vi "NiPxi6733.vi"() -> ()   [LabVIEW 2018, in "Visualization.lvlib" / "VisualizeFGen.lvclass"]
doc: "This VI listens for any measurement data associated with the provided PluginName and displays it to the user for analysis. The display is only suitable for data coming from the RoomAlert Plugin."
uses:
  VisualizeFGen.lvclass
  <vilib>/event_ctls.llb/usereventprio.ctl
  VisualizeBase/VisualizeBase_class/Requests/VisUserEventType.ctl
  <extravilib>/ChannelInstances/Tag-bool/Write With Abort.vi
  <extravilib>/ChannelInstances/Tag-bool/Read With Abort.vi
  <extravilib>/ChannelInstances/Tag-bool/Instantiate.vi
  <extravilib>/ChannelInstances/Tag-bool/EndpointRead.vi
  <vilib>/Utility/error.llb/Error Cluster From Error Code.vi
  <extravilib>/ChannelInstances/Tag-bool/Endpoint.vi
  <vilib>/ErrorRing/Error Ring.xnode
  <userlib>/NIST/NISTErrorLib/NISTErrorLib.lvlib
  <extravilib>/ChannelInstances/Tag-bool.lvlib
  TestClass/Test.lvclass
  VisualizeBase/VisualizeBase_class/VisualizeBase.lvclass
  FGen/FgenShared/FgenShared.lvlib
panel:
  in  "btnPause":bool=TRUE
  in  "ModuleID":i32
  in  "Log Data":bool
  in  "btnStop":bool
  in  "btnReset":bool
  in  "btnClearTest":bool
  out "WfrmGraph":waveform(dbl)[](graph)=[{"t0"=timestamp(3657200531.6397257 s since 1904-01-01), "dt"=1.0, "Y"=[46.19]}, {"t0"=timestamp(3657200531.6397257 s since 1904-01-01), "dt"=1.0, "Y"=[2.0]}, {"t0"=timestamp(3657200531.6397257 s since 1904-01-01), "dt"=1.0, "Y"=[60.0]}]
  out "ErrorArray":errorcluster[](array[cluster])
  in  "PluginName":string="Sensor.RoomAlert1"
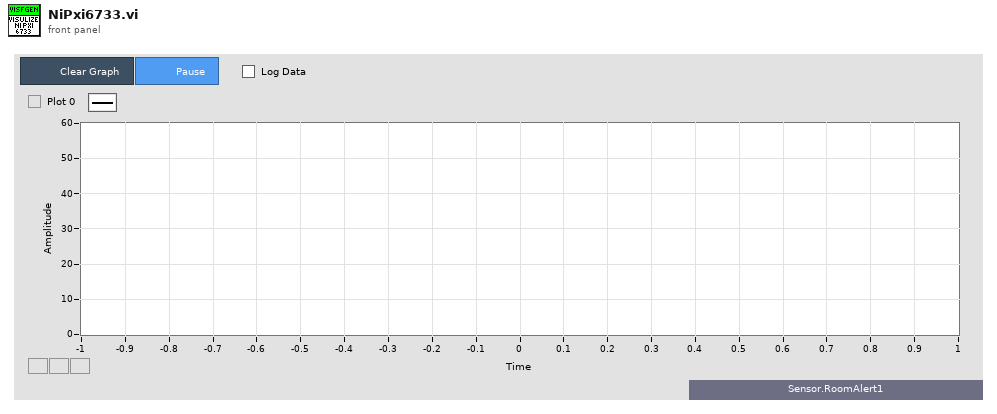
[diagram p1: front panel]
types:
  T1 = enum16{"open", "open or create", "create or replace", "create", "open (read-only)"}
  T2 = typedef "Visualization.lvlib/VisualizeBase.lvclass/VisRequestEvents.ctl" = cluster{"StopRequest":refnum<user-event>, "ResetRequest":refnum<user-event>, "FP Pop In or Out":refnum<user-event>}
  T3 = typedef "FgenShared.lvlib/clBroadcastEvents.ctl" = cluster{"DidInit":refnum<user-event>, "StatusUpdate":refnum<user-event>, "ErrorReport":refnum<user-event>, "DidStop":refnum<user-event>, "PathToINI":refnum<user-event>, "Channels":refnum<user-event>, "Function":refnum<user-event>, "Waveforms":refnum<user-event>, "Triggers":refnum<user-event>, "FunctionParams":refnum<user-event>, "FunctionArbs":refnum<user-event>, "FunctionSampleRate":refnum<user-event>}
  T4 = typedef "Visualization.lvlib/VisualizeBase.lvclass/VisUserEventType.ctl" = cluster{"BusIndex":i8, "Data":variant}
  T5 = typedef "usereventprio.ctl" = enum32{"high priority", "normal priority"}
  T6 = typedef "Tag-bool.lvlib/))Channel.ctl" = refnum<queue>
  T7 = typedef "sizeaction.ctl" = enum32{"Minimized", "Maximized", "Resized"}
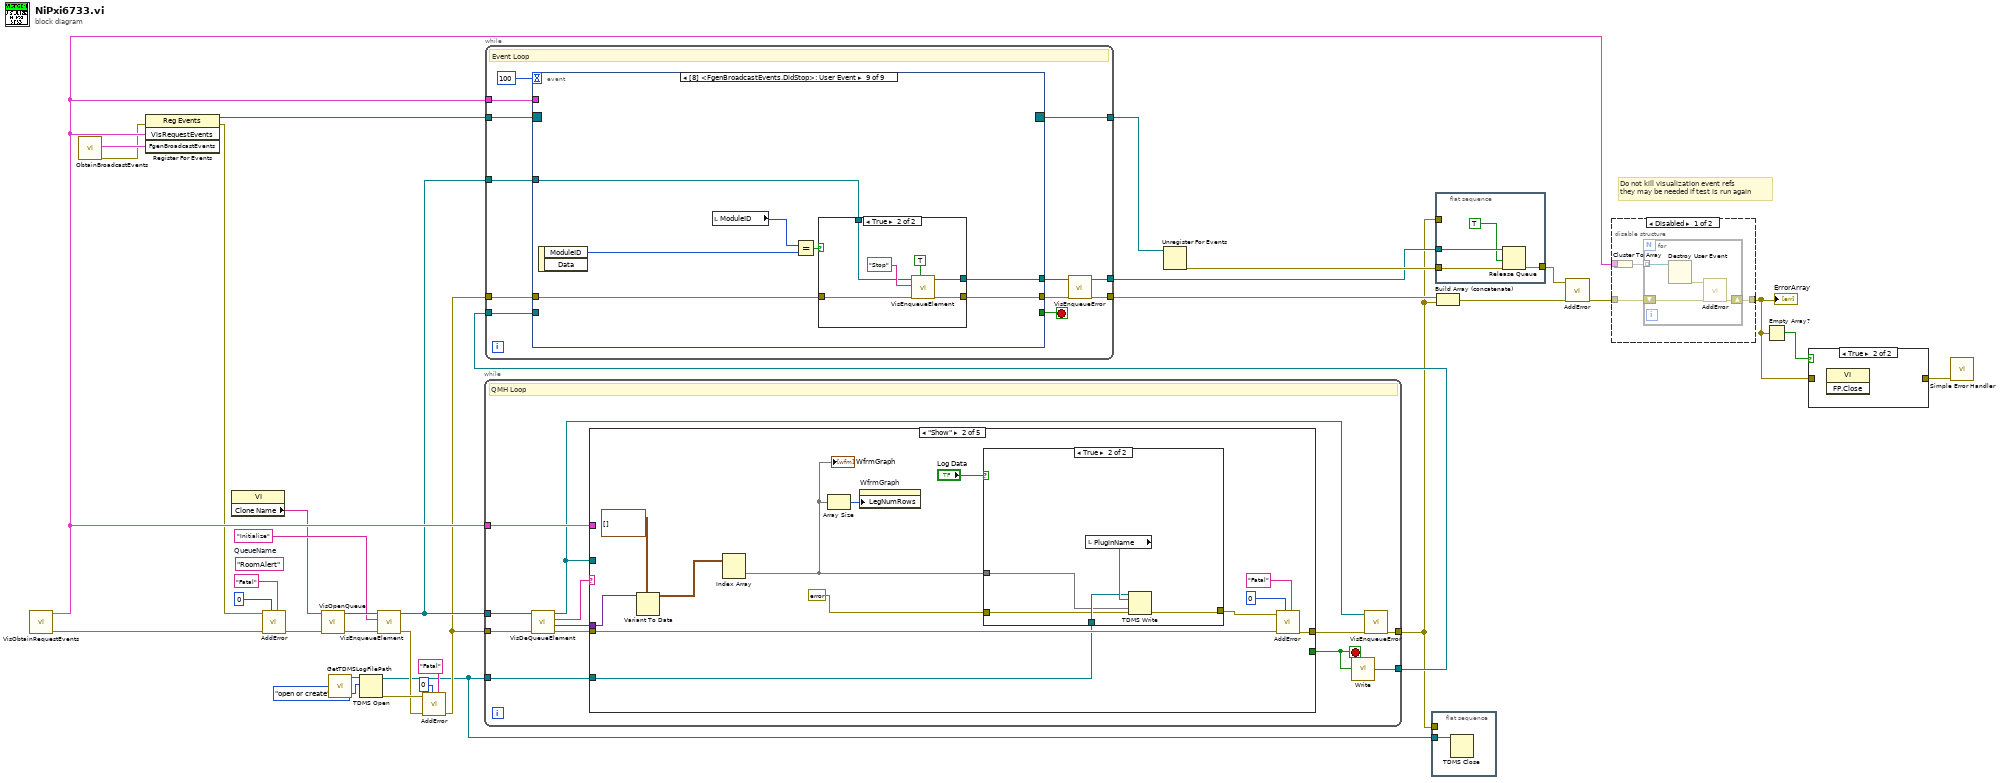
[diagram p0: block diagram]
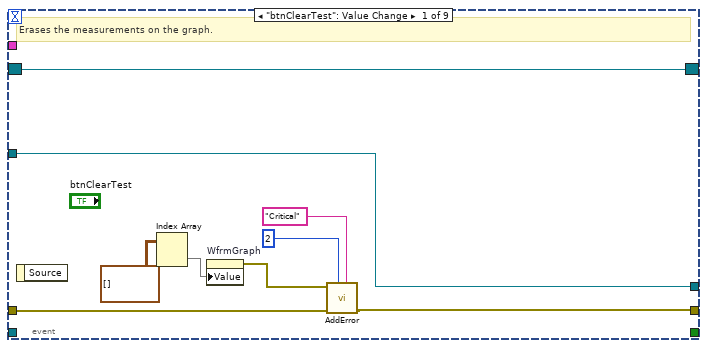
[diagram p3: hidden frame]
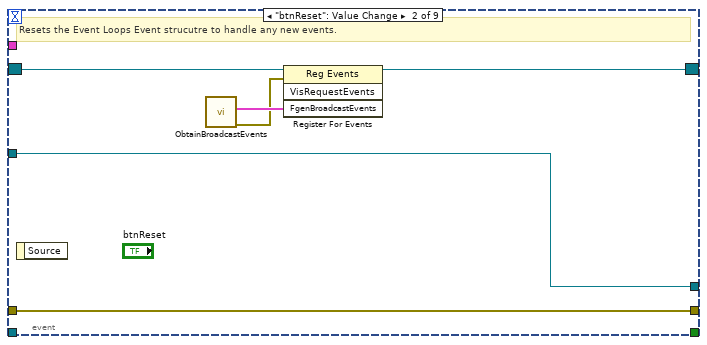
[diagram p4: hidden frame]
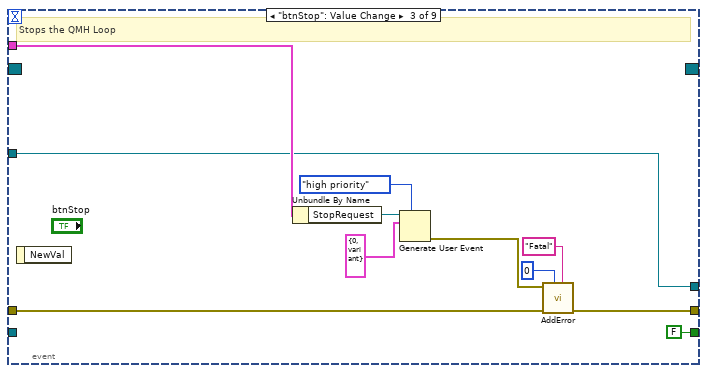
[diagram p5: hidden frame]
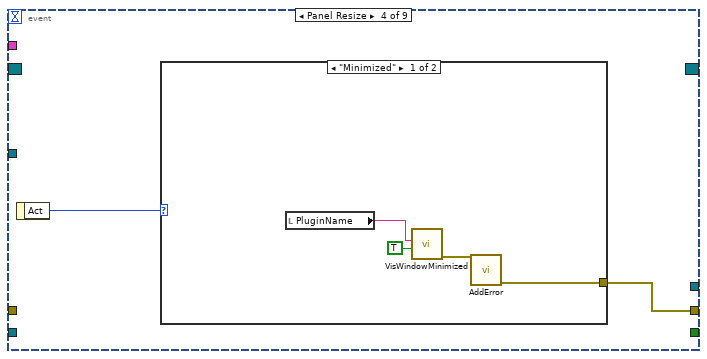
[diagram p6: hidden frame]
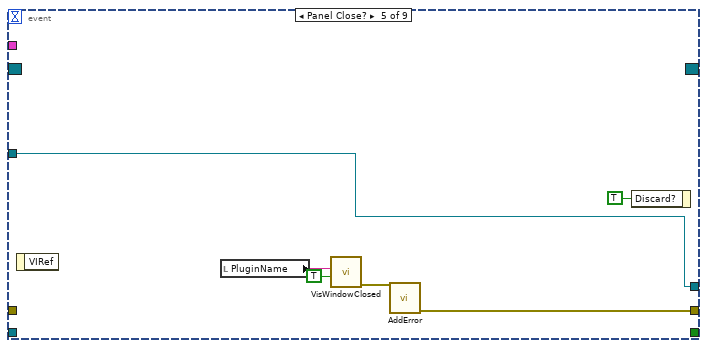
[diagram p8: hidden frame]
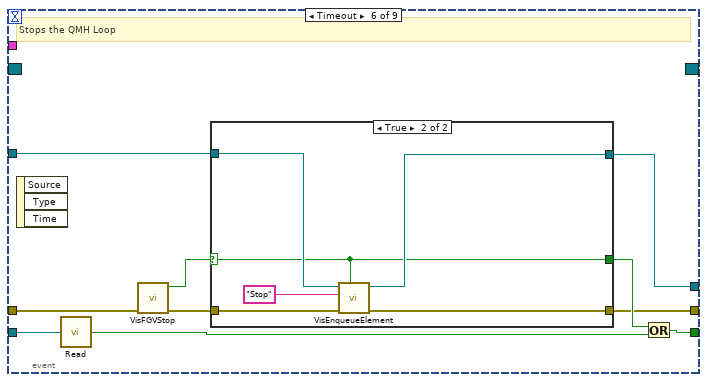
[diagram p9: hidden frame]
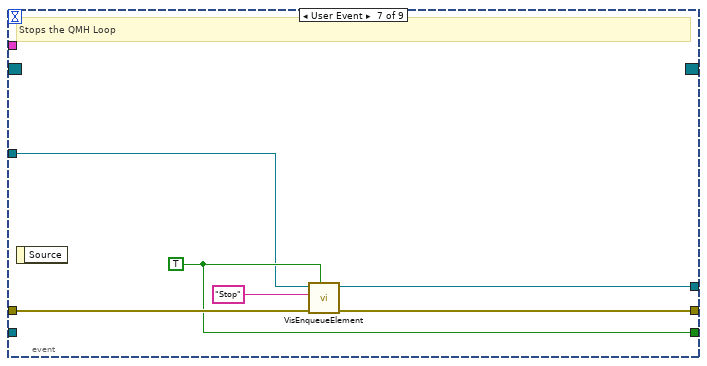
[diagram p11: hidden frame]
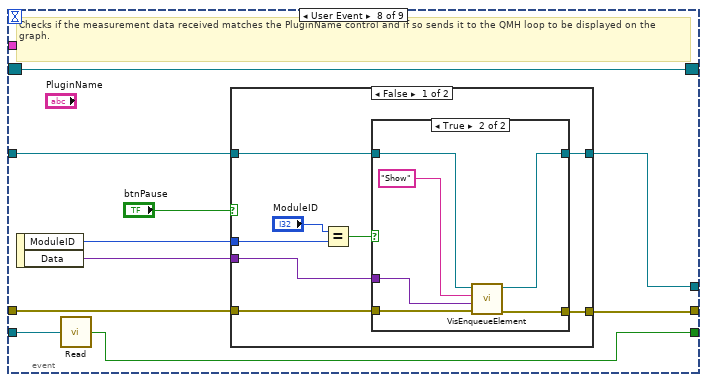
[diagram p12: hidden frame]
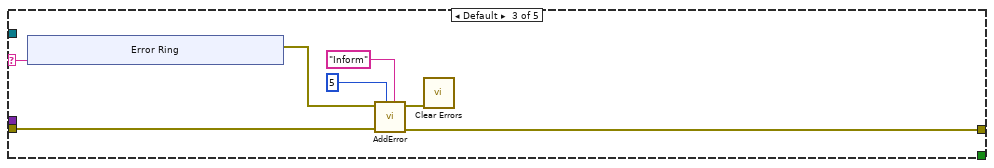
[diagram p18: hidden frame]
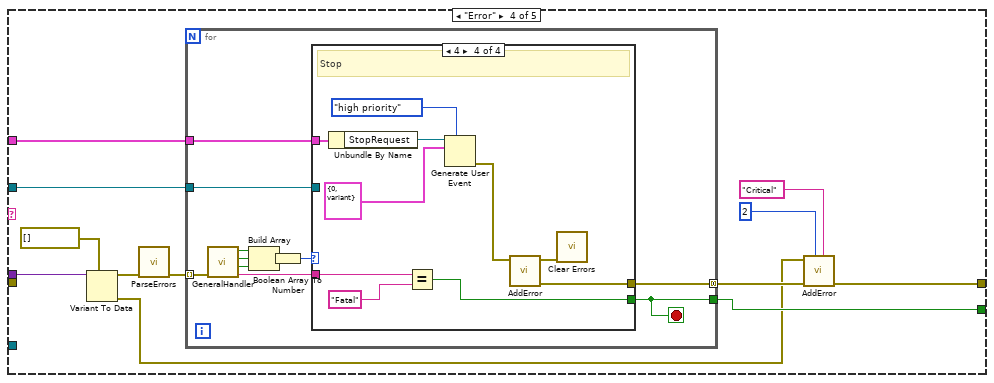
[diagram p19: hidden frame]
diagram:
  (unwired) "RoomAlert"  # QueueName
  # "Do not kill visualization event refs\nthey may be needed if test is run again"
  n1 = call "VisObtainRequestEvents.vi"() -> ("Error"=w25:errorcluster[], "VisRequestEvents"=w27:T2)  [unwired: 10 in]
  n2 = call "ObtainBroadcastEvents.vi"() -> ("error out"=w1:errorcluster, "FgenBroadcastEvents"=w2:T3)  [unwired: 10 in]
  n3 = register-events(error in=w1, w27, w2) -> (reference out=w34:refnum<event-registration>, error out=w24:errorcluster)  [unwired: 1 in]
  n4 = property class="VI"() -> ("Clone Name"=w12:string)  [unwired: 2 in, 2 out]
  n5 = call <userlib>:"AddError.vi"("Severity"="Fatal", "Priority"=u8 0, "ErrorArray In"=w25, "error in (no error)"=w24) -> ("ErrorArray Out"=w21:errorcluster[])  [unwired: 6 in, 1 out]
  n6 = call "VisOpenQueue.vi"("Error Array In"=w21, "QueueName"=w12) -> ("Error Array Out"=w19:errorcluster[], "queue out"=w20:refnum<queue>)  [unwired: 8 in]
  n7 = call "GetTDMSLogFilePath.vi"() -> ("TDMS Log File Path"=w11:path)  [unwired: 11 in]
  n8 = TDMS Open(10:T1."open or create" ("operation (0:open)"), 11:w11) -> (0:w8:errorcluster, 3:w4:refnum<k34>)  [unwired: 5 in]
  n9 = call "VisEnqueueElement.vi"("Error Array In"=w19, "Message"="Initialize", "queue in"=w20) -> ("Error Array Out"=w7:errorcluster[], "queue out"=w17:refnum<queue>)  [unwired: 7 in]
  n10 = call <userlib>:"AddError.vi"("Severity"="Fatal", "Priority"=u8 0, "ErrorArray In"=w7, "error in (no error)"=w8) -> ("ErrorArray Out"=w6:errorcluster[])  [unwired: 6 in, 1 out]
  n11 = while {
    tunnel: w6 -> [w40]
    tunnel: [w43] -> w3
    tunnel: w17 -> [w39]
    tunnel: w27 -> [w45]
    tunnel: [w36] -> w13
    tunnel: w4 -> [w35]
    stop <- w46 stop-if-true
    # "QMH Loop"
    n12 = call "VisDeQueueElement.vi"("Error Array In"=w40, "Queue In"=w39) -> ("Error Array Out"=w38:errorcluster[], "Data"=w41:variant, "Message"=w42:string, "Queue Out"=w37:refnum<queue>)  [unwired: 6 in]
    n13 = case shown="\"Show\"" w42 {
      selector: w42 -> [_ _ w73 _ _]
      tunnel: w41 -> [_ w56 _ w92 _]
      tunnel: w38 -> [w47 w59 w71 _ w119]
      tunnel: [w47 w60 w70 w82 w119] -> w44
      tunnel: [_ _ _ w88 TRUE] -> w46
      tunnel: w45 -> [_ _ _ w87 _]
      tunnel: w37 -> [_ _ _ w86 _]
      tunnel: w35 -> [_ w53 _ _ _]
      frame "Initialize" {
      }
      frame "Show" {
        n14 = Variant To Data(type=waveform(dbl)[][] [] ("data"), Variant=w56) -> (data=w50:waveform(dbl)[][])  [unwired: 1 in, 1 out]
        n15 = Index Array(array=w50) -> (element=w49:waveform(dbl)[])  [unwired: 2 in]
        "WfrmGraph" <- w49
        n16 = Array Size(array=w49) -> (size(s)=w52:i32)
        n17 = property on="WfrmGraph" class="WFGraph (strict)"("LegNumRows"=w52) -> ()  [unwired: 2 in, 2 out]
        n18 = case shown="True" "Log Data" {
          tunnel: errorcluster {"status"=FALSE, "code"=0, "source"=""} ("error out") -> [w61 w62]
          tunnel: [w61 w66] -> w55
          tunnel: w53 -> [_ w64]
          tunnel: w49 -> [_ w63]
          frame False {
          }
          frame True {
            n19 = local read "PluginName"() -> (w65:string)
            n20 = TDMS Write(0:w64, 5:w65, 9:w63, 11:w62) -> (15:w66:errorcluster)  [unwired: 2 in, 3 out]
          }
        }
        n21 = call <userlib>:"AddError.vi"("Severity"="Fatal" ("String"), "Priority"=u8 0, "ErrorArray In"=w59, "error in (no error)"=w55) -> ("ErrorArray Out"=w60:errorcluster[])  [unwired: 6 in, 1 out]
      }
      frame Default {
        n22 = xnode "Error Ring"("parameter 0"=w73) -> ("error out"=w72:errorcluster)
        n23 = call <userlib>:"AddError.vi"("Severity"="Inform" ("String"), "Priority"=u8 5, "ErrorArray In"=w71, "error in (no error)"=w72) -> ("ErrorArray Out"=w70:errorcluster[], "error out"=w69:errorcluster)  [unwired: 6 in]
        n24 = call <vilib>:"Clear Errors.vi"("error in (no error)"=w69) -> ()  [unwired: 5 in, 2 out]
      }
      frame "Error" {
        n25 = Variant To Data(type=errorcluster[] [], Variant=w92) -> (data=w90:errorcluster[], error out=w81:errorcluster)  [unwired: 1 in]
        n26 = call <userlib>:"ParseErrors.vi"("ErrorArray"=w90) -> ("ErrorArray"=w89:errorcluster[])  [unwired: 8 in, 2 out]
        n27 = for {
          tunnel: w89 -> [w103] mode=indexing
          tunnel: [w97] -> w83 mode=concatenating
          tunnel: [w95] -> w88
          tunnel: w87 -> [w94]
          tunnel: w86 -> [w93]
          stop <- w95 stop-if-true
          n28 = call <userlib>:"GeneralHandler.vi"("error in (no error)"=w103) -> ("Severity"=w96:string, "Stop"=w100:bool, "Abort"=w101:bool, "Continue"=w102:bool)  [unwired: 6 in, 1 out]
          n29 = Build Array(w102, w101, w100) -> (w99:bool[])
          n30 = Boolean Array To Number(Boolean array=w99) -> (number=w98:u32)
          n31 = case shown="4" w98 {
            tunnel: [_ _ w108 w117] -> w97
            tunnel: w96 -> [_ _ _ w110]
            tunnel: [_ _ _ w112] -> w95
            tunnel: w94 -> [_ _ _ w111]
            tunnel: w93 -> [_ _ w104 _]
            frame 0, Default {
              # "No Dialog"
            }
            frame 1 {
              # "Continue"
            }
            frame 2 {
              # "Abort, Flush Queue"
              n32 = Flush Queue(queue=w104) -> (error out=w107:errorcluster)  [unwired: 1 in, 2 out]
              n33 = call <userlib>:"AddError.vi"("Severity"="Critical" ("String"), "Priority"=u8 1, "error in (no error)"=w107) -> ("ErrorArray Out"=w108:errorcluster[])  [unwired: 7 in, 1 out]
            }
            frame 4 {
              # "Stop"
              n34 = Unbundle By Name(w111) -> ("StopRequest"=w118:refnum<user-event>)
              n35 = Equal?(x=w110, y="Fatal" ("x")) -> (x = y?=w112:bool)
              n36 = Generate User Event(priority (normal)=usereventprio."high priority", user event=w118, event data cluster=T4 {"BusIndex"=0, "Data"=variant} ("event data")) -> (error out=w116:errorcluster)  [unwired: 1 in, 1 out]
              n37 = call <userlib>:"AddError.vi"("error in (no error)"=w116) -> ("ErrorArray Out"=w117:errorcluster[], "error out"=w113:errorcluster)  [unwired: 9 in]
              n38 = call <vilib>:"Clear Errors.vi"("error in (no error)"=w113) -> ()  [unwired: 5 in, 2 out]
            }
          }
        }
        n39 = call <userlib>:"AddError.vi"("Severity"="Critical", "Priority"=u8 2, "ErrorArray In"=w83, "error in (no error)"=w81) -> ("ErrorArray Out"=w82:errorcluster[])  [unwired: 6 in, 1 out]
      }
      frame "Stop" {
      }
    }
    n40 = call <extravilib>:"Write.vi"("element"=w46) -> ("channel"=w36:T6)  [unwired: 1 out]
    n41 = call "VisEnqueueError.vi"("Error Array In"=w44, "Queue in"=w37) -> ("Error Array Out"=w43:errorcluster[])  [unwired: 8 in, 1 out]
  }
  n42 = while {
    tunnel: w34 -> [w132]
    tunnel: [w126] -> w32
    tunnel: [w130] -> w33
    tunnel: w27 -> [w129]
    tunnel: w6 -> [w128]
    tunnel: w17 -> [w127]
    tunnel: [w123] -> w16
    tunnel: w13 -> [w121]
    stop <- w131 stop-if-true
    # "Event Loop"
    n43 = event shown="[8] <FgenBroadcastEvents.DidStop>: User Event" {
      selector: w132 -> [w136 w147 _ _ _ _ _ w201 _]
      dyn-events: [w136 w146 _ _ _ _ _ w201 _] -> w130
      timeout: 100 -> [_ _ _ _ _ _ _ _ _]
      tunnel: [_ _ FALSE ("Priority? (F)") _ _ w171 w192 w199 _] -> w131
      tunnel: [w138 w145 w151 w159 w166 w173 w194 w203 w230] -> w125
      tunnel: w129 -> [_ _ w150 _ _ _ _ _ _]
      tunnel: w128 -> [w139 w145 w158 _ _ w176 w195 w204 w224]
      tunnel: w127 -> [w135 w144 w148 _ w165 w175 w190 w205 w228]
      tunnel: [w135 w144 w148 _ w165 w174 w193 w202 w229] -> w124
      tunnel: w121 -> [_ _ _ _ _ w180 _ w200 _]
      event "btnClearTest": Value Change {
        # "Erases the measurements on the graph."
        n44 = event-data() -> ()  [unwired: 1 in, 1 out]
        n45 = Index Array(array=waveform(dbl)[][] [] ("History Data")) -> (element=w133:waveform(dbl)[])  [unwired: 2 in]
        n46 = property on="WfrmGraph" class="WFGraph (strict)"("Value"=w133) -> (error out=w137:errorcluster)  [unwired: 2 in, 1 out]
        n47 = call <userlib>:"AddError.vi"("Severity"="Critical", "Priority"=u8 2, "ErrorArray In"=w139, "error in (no error)"=w137) -> ("ErrorArray Out"=w138:errorcluster[])  [unwired: 6 in, 1 out]
      }
      event "btnReset": Value Change {
        # "Resets the Event Loops Event strucutre to handle any new events."
        n48 = event-data() -> ()  [unwired: 1 in, 1 out]
        n49 = call "ObtainBroadcastEvents.vi"() -> ("error out"=w142:errorcluster, "FgenBroadcastEvents"=w143:T3)  [unwired: 10 in]
        n50 = register-events(reference=w147, error in=w142, w143) -> (reference out=w146:refnum<event-registration>)  [unwired: 1 in, 1 out]
      }
      event "btnStop": Value Change {
        # "Stops the QMH Loop"
        n51 = event-data() -> ()  [unwired: 1 in, 1 out]
        n52 = Unbundle By Name(w150) -> ("StopRequest"=w156:refnum<user-event>)
        n53 = Generate User Event(priority (normal)=usereventprio."high priority", user event=w156, event data cluster=T4 {"BusIndex"=0, "Data"=variant} ("event data")) -> (error out=w157:errorcluster)  [unwired: 1 in, 1 out]
        n54 = call <userlib>:"AddError.vi"("Severity"="Fatal" ("String"), "Priority"=u8 0, "ErrorArray In"=w158, "error in (no error)"=w157) -> ("ErrorArray Out"=w151:errorcluster[])  [unwired: 6 in, 1 out]
      }
      event Panel Resize {
        n55 = event-data() -> ("Act"=w160:T7)  [unwired: 1 in]
        n56 = case shown="\"Minimized\"" w160 {
          tunnel: [w161 _] -> w159
          frame "Minimized" {
            n57 = local read "PluginName"() -> (w163:string)
            n58 = call "VisWindowMinimized.vi"("Window Minimized?"=TRUE ("Window Minimized or Clozed?"), "Module Name"=w163) -> ("error out"=w164:errorcluster)  [unwired: 9 in]
            n59 = call <userlib>:"AddError.vi"("error in (no error)"=w164) -> ("ErrorArray Out"=w161:errorcluster[])  [unwired: 9 in, 1 out]
          }
          frame "Maximized", Default {
          }
        }
      }
      event Panel Close? {
        n60 = event-data() -> ()  [unwired: 1 in, 1 out]
        n61 = local read "PluginName"() -> (w167:string)
        n62 = call "VisWindowClosed.vi"("Window Closed?"=TRUE ("Window Minimized or Clozed?"), "Module Name"=w167) -> ("error out"=w169:errorcluster)  [unwired: 9 in]
        n63 = call <userlib>:"AddError.vi"("error in (no error)"=w169) -> ("ErrorArray Out"=w166:errorcluster[])  [unwired: 9 in, 1 out]
        n64 = event-data("Discard?"=TRUE) -> ()  [unwired: 1 in, 1 out]
      }
      event Timeout {
        # "Stops the QMH Loop"
        n65 = event-data() -> ()  [unwired: 1 in, 3 out]
        n66 = call <extravilib>:"Read.vi"("channel"=w180) -> ("element"=w172:bool)  [unwired: 1 in, 1 out]
        n67 = call "VisFGVStop.vi"("Error In"=w176) -> ("Error Out"=w178:errorcluster[], "Value"=w179:bool)  [unwired: 9 in]
        n68 = case shown="True" w179 {
          selector: w179 -> [w181 w184]
          tunnel: [w183 w187] -> w173
          tunnel: w178 -> [w183 w188]
          tunnel: w175 -> [w182 w186]
          tunnel: [w182 w185] -> w174
          tunnel: [w181 w184] -> w177
          frame False {
          }
          frame True {
            n69 = call "VisEnqueueElement.vi"("Priority? (F)"=w184, "Error Array In"=w188, "Message"="Stop", "queue in"=w186) -> ("Error Array Out"=w187:errorcluster[], "queue out"=w185:refnum<queue>)  [unwired: 6 in]
          }
        }
        n70 = Or(x=w177, y=w172) -> (x .or. y?=w171:bool)
      }
      event User Event {
        w192 = TRUE ("Priority? (F)")
        # "Stops the QMH Loop"
        n71 = event-data() -> ()  [unwired: 1 in, 1 out]
        n72 = call "VisEnqueueElement.vi"("Priority? (F)"=w192, "Error Array In"=w195, "Message"="Stop", "queue in"=w190) -> ("Error Array Out"=w194:errorcluster[], "queue out"=w193:refnum<queue>)  [unwired: 6 in]
      }
      event User Event {
        # "Checks if the measurement data received matches the PluginName control and if so sends it to the QMH loop to be displayed on the graph."
        n73 = event-data() -> ("ModuleID"=w197:i32, "Data"=w198:variant)  [unwired: 1 in]
        n74 = call <extravilib>:"Read.vi"("channel"=w200) -> ("element"=w199:bool)  [unwired: 1 in, 1 out]
        n75 = case shown="False" "btnPause" {
          tunnel: w205 -> [w213 w223]
          tunnel: w204 -> [w212 w222]
          tunnel: [w211 w222] -> w203
          tunnel: [w210 w223] -> w202
          tunnel: w198 -> [w208 _]
          tunnel: w197 -> [w207 _]
          frame False {
            n76 = Equal?(x="ModuleID", y=w207) -> (x = y?=w209:bool)
            n77 = case shown="True" w209 {
              tunnel: [w214 w220] -> w211
              tunnel: w213 -> [w215 w219]
              tunnel: w212 -> [w214 w221]
              tunnel: [w215 w218] -> w210
              tunnel: w208 -> [_ w216]
              frame False {
              }
              frame True {
                n78 = call "VisEnqueueElement.vi"("Error Array In"=w221, "Data"=w216, "Message"="Show", "queue in"=w219) -> ("Error Array Out"=w220:errorcluster[], "queue out"=w218:refnum<queue>)  [unwired: 6 in]
              }
            }
          }
          frame True {
          }
        }
      }
      event User Event {
        n79 = event-data() -> ("ModuleID"=w225:i32)  [unwired: 1 in, 1 out]
        n80 = local read "ModuleID"() -> (w227:i32)
        n81 = Equal?(x=w227, y=w225) -> (x = y?=w226:bool)
        n82 = case shown="True" w226 {
          tunnel: [w231 w236] -> w230
          tunnel: [w232 w235] -> w229
          tunnel: w228 -> [w232 w234]
          tunnel: w224 -> [w231 w233]
          frame False {
          }
          frame True {
            n83 = call "VisEnqueueElement.vi"("Priority? (F)"=TRUE, "Error Array In"=w233, "Message"="Stop", "queue in"=w234) -> ("Error Array Out"=w236:errorcluster[], "queue out"=w235:refnum<queue>)  [unwired: 6 in]
          }
        }
      }
    }
    n84 = call "VisEnqueueError.vi"("Error Array In"=w125, "Queue in"=w124) -> ("Error Array Out"=w126:errorcluster[], "Queue out"=w123:refnum<queue>)  [unwired: 8 in]
  }
  n85 = Unregister For Events(event registration refnum=w33) -> (error out=w31:errorcluster)  [unwired: 1 in]
  n86 = flat-sequence {
    tunnel: w4 -> [w239]
    tunnel: w3 -> [_]
    frame #0 {
      n87 = TDMS Close(11:w239) -> ()  [unwired: 1 in, 2 out]
    }
  }
  n88 = flat-sequence {
    tunnel: w31 -> [w243]
    tunnel: [w242] -> w29
    tunnel: w16 -> [w241]
    tunnel: w3 -> [_]
    frame #0 {
      n89 = Release Queue(queue=w241, force destroy? (F)=TRUE, error in (no error)=w243) -> (error out=w242:errorcluster)  [unwired: 2 out]
    }
  }
  n90 = Build Array (concatenate)(w32, w3) -> (w30:errorcluster[])
  n91 = call <userlib>:"AddError.vi"("ErrorArray In"=w30, "error in (no error)"=w29) -> ("ErrorArray Out"=w28:errorcluster[])  [unwired: 8 in, 1 out]
  n92 = disable-structure shown="Disabled" {
    disable-tunnel: w28 -> [w246 w252]
    disable-tunnel: w27 -> [w245 _]
    disable-tunnel: [w244 w252] -> w15
    frame Disabled {
      n93 = Cluster To Array(cluster=w245) -> (array=w247:refnum<user-event>[])
      n94 = for {
        tunnel: w247 -> [w251] mode=indexing
        shift-right: [w250] -> w244
        shift-left: w246 -> [w249]
        n95 = Destroy User Event(user event=w251) -> (error out=w248:errorcluster)  [unwired: 1 in]
        n96 = call <userlib>:"AddError.vi"("ErrorArray In"=w249, "error in (no error)"=w248) -> ("ErrorArray Out"=w250:errorcluster[])  [unwired: 8 in, 1 out]
      }
    }
    frame Enabled {
    }
  }
  "ErrorArray" <- w15
  n97 = Empty Array?(array=w15) -> (empty?=w26:bool)
  n98 = case shown="True" w26 {
    tunnel: [w253 _] -> w14
    tunnel: w15 -> [w254 _]
    frame False {
      n99 = Merge Errors(w254) -> (w253:errorcluster)
    }
    frame True {
      n100 = invoke class="VI" method="FP.Close"() -> ()  [unwired: 3 in, 3 out]
    }
  }
  n101 = call <vilib>:"Simple Error Handler.vi"("error in (no error)"=w14) -> ()  [unwired: 4 in, 5 out]
